vi "Pre-Build VI - Run Unit Tests.vi"(8 "error in (no error)":errorcluster) -> (0 "error out":errorcluster, 1 "VIs without test coverage":string[](array[string]), 2 "error type":enum16{"fatal", "non-fatal", "warning"}(ring))   [LabVIEW 2009]
uses:
  <userlib>/_OpenG.lib/array/array.llb/Empty 1D Array (String)__ogtk.vi
  <userlib>/_OpenG.lib/array/array.llb/Filter 1D Array (String)__ogtk.vi
panel:
  in  "type specifier VI Refnum (for type only)":refnum<vi>
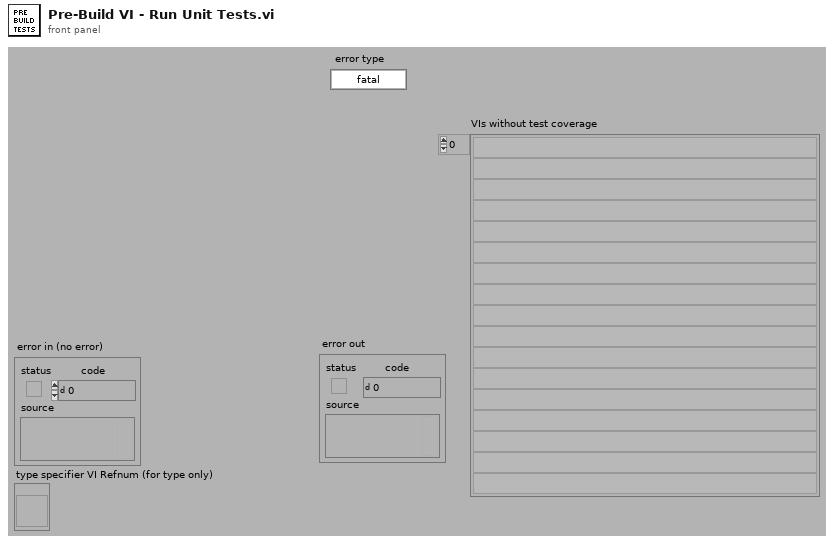
[diagram p1: front panel]
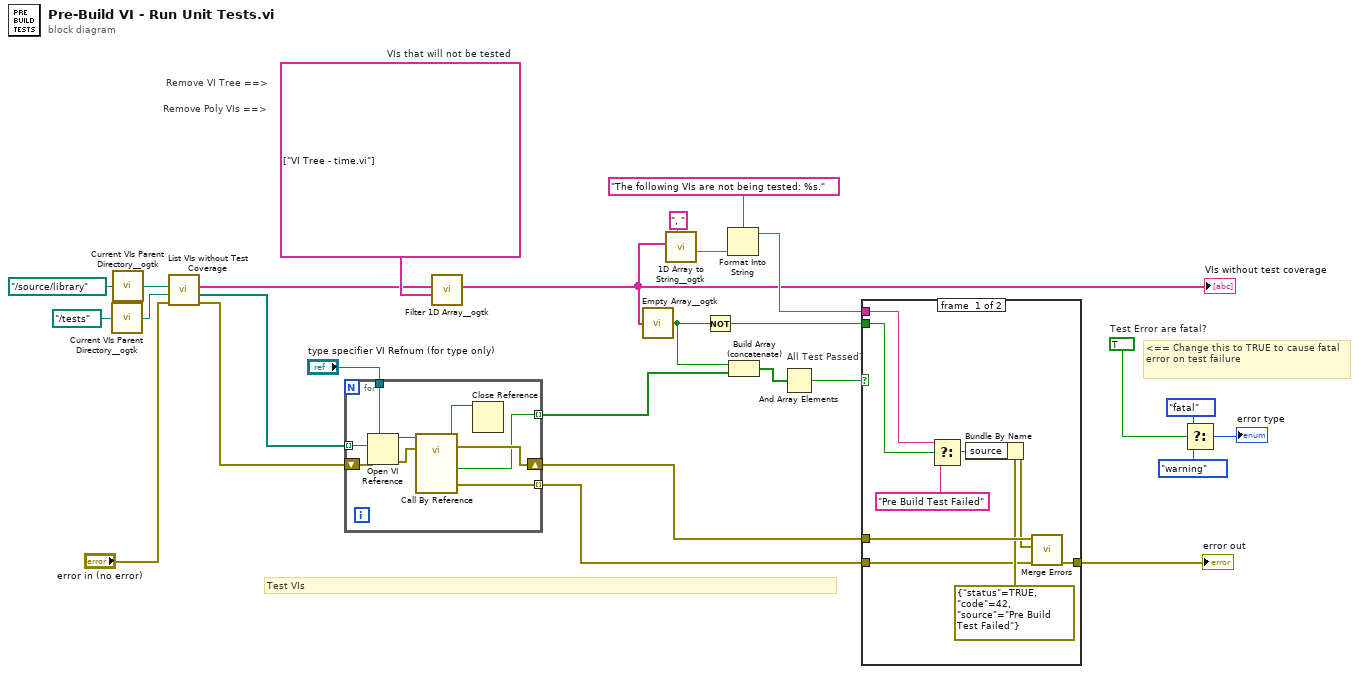
[diagram p0: block diagram]
diagram:
  w13 = TRUE  # Test Error are fatal?
  w25 = string[] ["VI Tree - time.vi"]  # VIs that will not be tested
  # "<== Change this to TRUE to cause fatal error on test failure"
  # "Remove Poly VIs ==>"
  # "Remove VI Tree ==>"
  # "All Test Passed?"
  # "Test VIs"
  n1 = call <userlib>:"Current VIs Parent Directory__ogtk.vi"("Relative path (.)"=path "../tests") -> ("Parent Directory (+ Relative)"=w8:path)  [unwired: 4 in]
  n2 = call <userlib>:"Current VIs Parent Directory__ogtk.vi"("Relative path (.)"=path "../source/library") -> ("Parent Directory (+ Relative)"=w17:path)  [unwired: 4 in]
  n3 = call "List VIs without Test Coverage.vi"("error in (no error)"="error in (no error)", "Tests Root"=w8, "Source Root"=w17) -> ("error out"=w4:errorcluster, "Test VIs"=w7:path[], "VIs without test coverage"=w24:string[])  [unwired: 6 in]
  n4 = for {
    tunnel: w7 -> [w36] mode=indexing
    tunnel: "type specifier VI Refnum (for type only)" -> [w35]
    shift-right: [w32] -> w5
    shift-left: w4 -> [w31]
    tunnel: [w30] -> w3 mode=indexing
    tunnel: [w28] -> w2 mode=indexing
    n5 = Open VI Reference(type specifier VI Refnum (for type only)=w35, vi path=w36, error in (no error)=w31) -> (vi reference=w34:refnum<vi>, error out=w33:errorcluster)  [unwired: 3 in]
    n6 = call-by-ref "?"(reference=w34, error in=w33) -> (reference out=w29:refnum<vi>, error out=w32:errorcluster, 0:"error out"=w28:errorcluster, "pass"=w30:bool)  [unwired: 10 in]
    n7 = Close Reference(reference=w29) -> ()  [unwired: 1 in, 1 out]
  }
  n8 = call-poly <userlib>:"Filter 1D Array__ogtk.vi"("items to filter"=w25, "array"=w24) -> ("filtered array"=w1:string[])  [unwired: 4 in, 1 out]
  "VIs without test coverage" <- w1
  n9 = call-poly <userlib>:"Empty Array__ogtk.vi"("Array"=w1) -> ("Empty Array?"=w19:bool)  [unwired: 8 in]
  n10 = call <userlib>:"1D Array to String__ogtk.vi"("delimiter (Tab)"=", ", "Array of Strings"=w1) -> ("delimited string"=w22:string)  [unwired: 9 in]
  n11 = Not(x=w19) -> (.not. x?=w18:bool)
  n12 = Format Into String(format string="The following VIs are not being tested: %s.", w22) -> (resulting string=w20:string)  [unwired: 2 in, 1 out]
  n13 = Build Array (concatenate)(w19, w3) -> (w27:bool[])
  n14 = And Array Elements(Boolean array=w27) -> (logical AND=w26:bool)
  n15 = case shown="False" w26 {
    tunnel: w5 -> [w45 w46]
    tunnel: [w44 w46] -> w15
    tunnel: w18 -> [w43 _]
    tunnel: w20 -> [w42 _]
    tunnel: w2 -> [w37 _]
    frame #0 {
      n16 = Select(t=w42, s=w43, f="Pre Build Test Failed" ("source")) -> (s? t:f=w40:string)
      n17 = Bundle By Name(cluster=errorcluster {"status"=TRUE, "code"=42, "source"="Pre Build Test Failed"} ("error out"), "source"=w40) -> (w39:errorcluster)
      n18 = call <vilib>:"Merge Errors.vi"("error array in"=w37, "error in 2 (no error)"=w39, "error in 1 (no error)"=w45) -> ("error out"=w44:errorcluster)  [unwired: 4 in]
    }
    frame #1 {
    }
  }
  "error out" <- w15
  n19 = Select(t=enum16{"fatal", "non-fatal", "warning"}."fatal" ("error type"), s=w13, f=enum16{"fatal", "non-fatal", "warning"}."warning" ("error type")) -> (s? t:f=→"error type":enum16{"fatal", "non-fatal", "warning"})
